vi "OxITC503 _VISA_ Close.vi"(1 "error in (no error)":errorcluster, 2 "VISA session":refnum<visa-resource-name>="GPIB::2") -> (0 "error out":errorcluster)   [LabVIEW 2013]
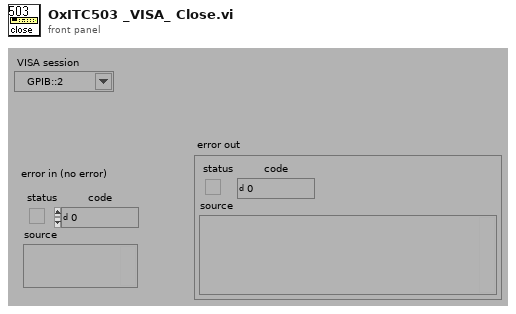
[diagram p1: front panel]
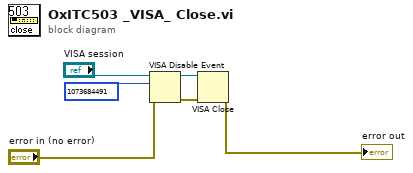
[diagram p0: block diagram]
diagram:
  n1 = VISA Disable Event(8:"error in (no error)", 10:u32 1073684491 ("event type"), 11:"VISA session") -> (0:w4:errorcluster, 3:w5:refnum<visa-resource-name>)  [unwired: 1 in]
  n2 = VISA Close(VISA resource name=w5, error in (no error)=w4) -> (error out=→"error out":errorcluster)
